vi "deployment tool.vi"(7 "current pcfg path":path, 8 "error in":errorcluster, 11 "root":refnum<data-value>) -> (0 "error out":errorcluster)   [LabVIEW 2013, in "PL Framework Configuration Tool.lvlib"]
uses:
  PL Framework Configuration Tool.lvlib
  <vilib>/NI/Configuration Framework/Node/NISE_CEF_Node.lvclass
  Classes/Systems/Systems.lvclass
  <vilib>/NI/Configuration Framework/Node/NISE_CEF_Node.lvclass/NISE_CEF_Node.ctl
  Classes/Targets/Targets.lvclass
  Framework Configuration Classes/target configuration/PL_Target Configuration.lvclass
  deployment configuration.ctl
  Classes/TBM Configuration Node/deployment configuration.ctl
  Classes/TBM Configuration Node/TBM Configuration Node.lvclass
  Framework Configuration Classes/target configuration/PL_Target Configuration.lvclass/PL_Target Configuration.ctl
  <vilib>/NI/Configuration Framework/Node/ReadChildren.vi
  Framework Configuration Classes/target configuration/Read Config Path.vi
  <vilib>/NI/Configuration Framework/serializable configuration/NISE_CEF_serializable configuration.lvclass
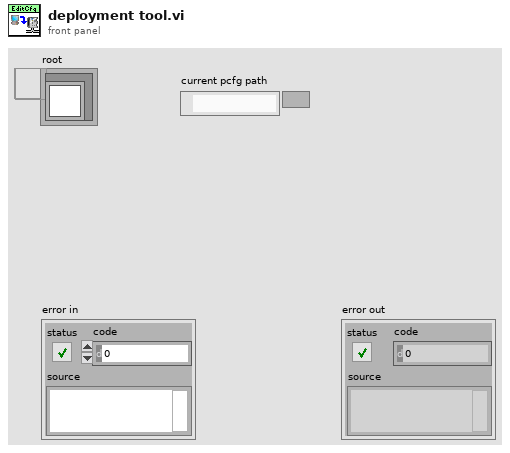
[diagram p1: front panel]
types:
  T1 = typedef "NISE_CEF_Node.lvclass/NodeRef.ctl" = refnum<data-value>
  T2 = typedef "PL Framework Configuration Tool.lvlib/TBM Configuration Node.lvclass/deployment configuration.ctl" = cluster{"local path":path, "remote path (relative to root)":path}
  T3 = typedef "PL Framework Configuration Tool.lvlib/deployment configuration.ctl" = cluster{"Target Configuration":refnum<class "PL_Target Configuration.lvclass">, "files":T2[], "all nodes":refnum<data-value>[]}
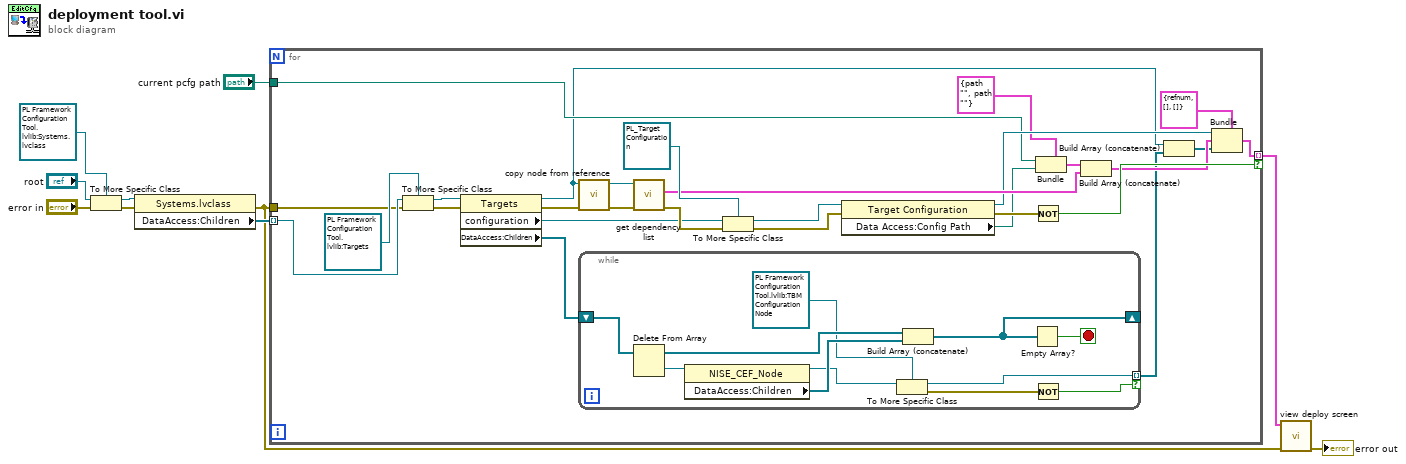
[diagram p0: block diagram]
diagram:
  n1 = To More Specific Class(target class=refnum<data-value> refnum, reference="root", error in="error in") -> (specific class reference=w8:refnum<data-value>, error out=w7:errorcluster)
  n2 = property class="Systems.lvclass"(reference=w8, error in=w7) -> (error out=w4:errorcluster, "DataAccess:Children"=w6:T1[])  [unwired: 1 out]
  n3 = for {
    tunnel: w6 -> [w38] mode=indexing
    tunnel: w4 -> [w36]
    tunnel: [w25] -> w5 mode=indexing if=w24
    tunnel: "current pcfg path" -> [w16]
    n4 = To More Specific Class(target class=refnum<data-value> refnum, reference=w38, error in=w36) -> (specific class reference=w34:refnum<data-value>, error out=w35:errorcluster)
    n5 = property class="Targets"(reference=w34, error in=w35) -> (reference out=w13:refnum<data-value>, error out=w32:errorcluster, "configuration"=w29:refnum<class "NISE_CEF_serializable configuration.lvclass">, "DataAccess:Children"=w14:T1[])
    n6 = call "copy node from reference.vi"("error in"=w32, "TBM node dvr"=w13) -> ("error out"=w31:errorcluster, "TBM node value"=w30:refnum<class "TBM Configuration Node.lvclass">)  [unwired: 8 in]
    n7 = while {
      shift-right: [w45] -> _
      shift-left: w14 -> [w49]
      tunnel: [w41] -> w12 mode=indexing if=w39
      stop <- w46 stop-if-true
      n8 = Delete From Array(array=w49) -> (deleted portion=w48:T1, array with subset deleted=w47:T1[])  [unwired: 2 in]
      n9 = property class="NISE_CEF_Node"(reference=w48) -> (reference out=w43:T1, "DataAccess:Children"=w44:T1[])  [unwired: 1 in, 1 out]
      n10 = To More Specific Class(target class=refnum<data-value> refnum, reference=w43) -> (specific class reference=w41:refnum<data-value>, error out=w40:errorcluster)  [unwired: 1 in]
      n11 = Build Array (concatenate)(w47, w44) -> (w45:T1[])
      n12 = Empty Array?(array=w45) -> (empty?=w46:bool)
      n13 = Not(x=w40) -> (.not. x?=w39:bool)
    }
    n14 = call-dynamic "get dependency list.vi"("error in"=w31, "TBM Configuration Node in"=w30) -> ("error out"=w33:errorcluster, "files"=w27:T2[])  [unwired: 7 in, 1 out]
    n15 = To More Specific Class(target class=refnum<class "PL_Target Configuration.lvclass"> refnum ("Target Configuration"), reference=w29, error in=w33) -> (specific class reference=w21:refnum<class "PL_Target Configuration.lvclass">, error out=w26:errorcluster)
    n16 = property class="Target Configuration"(reference=w21, error in=w26) -> (reference out=w20:refnum<class "PL_Target Configuration.lvclass">, error out=w22:errorcluster, "Data Access:Config Path"=w15:path)
    n17 = Not(x=w22) -> (.not. x?=w24:bool)
    n18 = Bundle(cluster=T2 {"local path"=path "", "remote path (relative to root)"=path ""} ("deployment configuration"), "local path"=w16, "remote path (relative to root)"=w15) -> (w18:T2)
    n19 = Build Array (concatenate)(w18, w27) -> (w19:T2[])
    n20 = Build Array (concatenate)(w13, w12) -> (w11:refnum<data-value>[])
    n21 = Bundle(cluster=T3 {"Target Configuration"=refnum, "files"=[], "all nodes"=[]}, "Target Configuration"=w20, "files"=w19, "all nodes"=w11) -> (w25:T3)
  }
  n22 = call "view deploy screen.vi"("error in"=w4, "deployment configuration"=w5) -> ("error out"=→"error out":errorcluster)  [unwired: 9 in]
